vi "RichToFlatcif_manager_ClockConversion.vi"(5 "OutputClusterType":T1, 11 "InputCluster":T3) -> (3 "OutputCluster":T1)   [LabVIEW 2021, in "CIF_PluginLoader_server.lvlib"]
uses:
  CIF_PluginLoader_server.lvlib
  cif_manager_ClockConversion.ctl
  cif_manager_TimePair.ctl
  cif_manager_ClockConversion_Flat.ctl
  cif_manager_TimePair_Flat.ctl
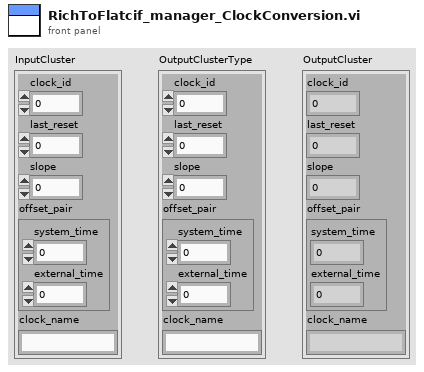
[diagram p1: front panel]
types:
  T1 = typedef "CIF_PluginLoader_server.lvlib/cif_manager_ClockConversion_Flat.ctl" = cluster{"clock_id":u32, "last_reset":i64, "slope":dbl, "offset_pair":T2, "clock_name":string}
  T2 = typedef "CIF_PluginLoader_server.lvlib/cif_manager_TimePair_Flat.ctl" = cluster{"system_time":i64, "external_time":i64}
  T3 = typedef "CIF_PluginLoader_server.lvlib/cif_manager_ClockConversion.ctl" = cluster{"clock_id":u32, "last_reset":i64, "slope":dbl, "offset_pair":T4, "clock_name":string}
  T4 = typedef "CIF_PluginLoader_server.lvlib/cif_manager_TimePair.ctl" = cluster{"system_time":i64, "external_time":i64}
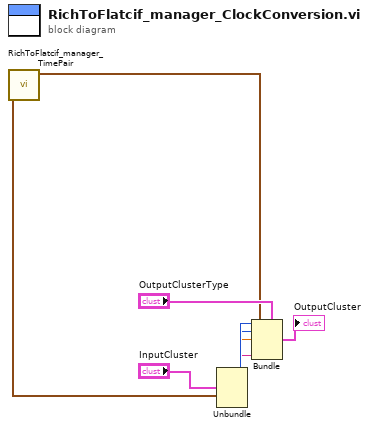
[diagram p0: block diagram]
diagram:
  n1 = Unbundle "Unbundle"("InputCluster") -> ("clock_id"=w6:u32, "last_reset"=w5:i64, "slope"=w4:dbl, "offset_pair"=w3:T4, "clock_name"=w1:string)
  n2 = call "RichToFlatcif_manager_TimePair.vi"("InputCluster"=w3) -> ("OutputCluster"=w2:T2)  [unwired: 10 in]
  n3 = Bundle "Bundle"(cluster="OutputClusterType", "clock_id"=w6, "last_reset"=w5, "slope"=w4, "offset_pair"=w2, "clock_name"=w1) -> (→"OutputCluster":T1)
